vi "同步显示.vi"(8 "error in (no error)":errorcluster caption="错误输入（无错误）", 11 "程序 输入":refnum<class "程序.lvclass">) -> (0 "error out":errorcluster caption="错误输出", 3 "程序 输出":refnum<class "程序.lvclass">)   [LabVIEW 2018, in "程序.lvclass"]
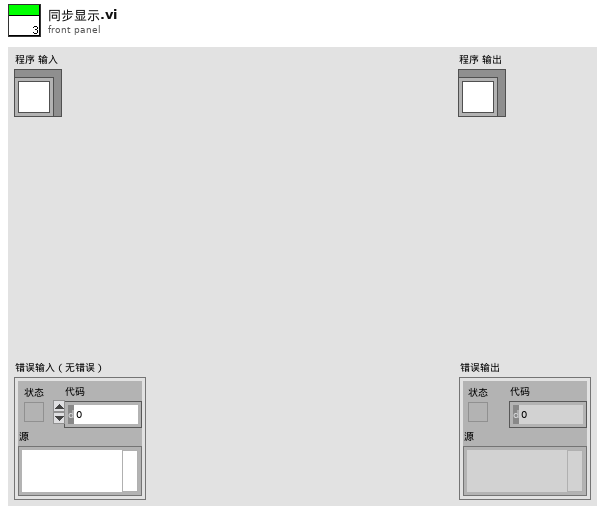
[diagram p1: front panel]
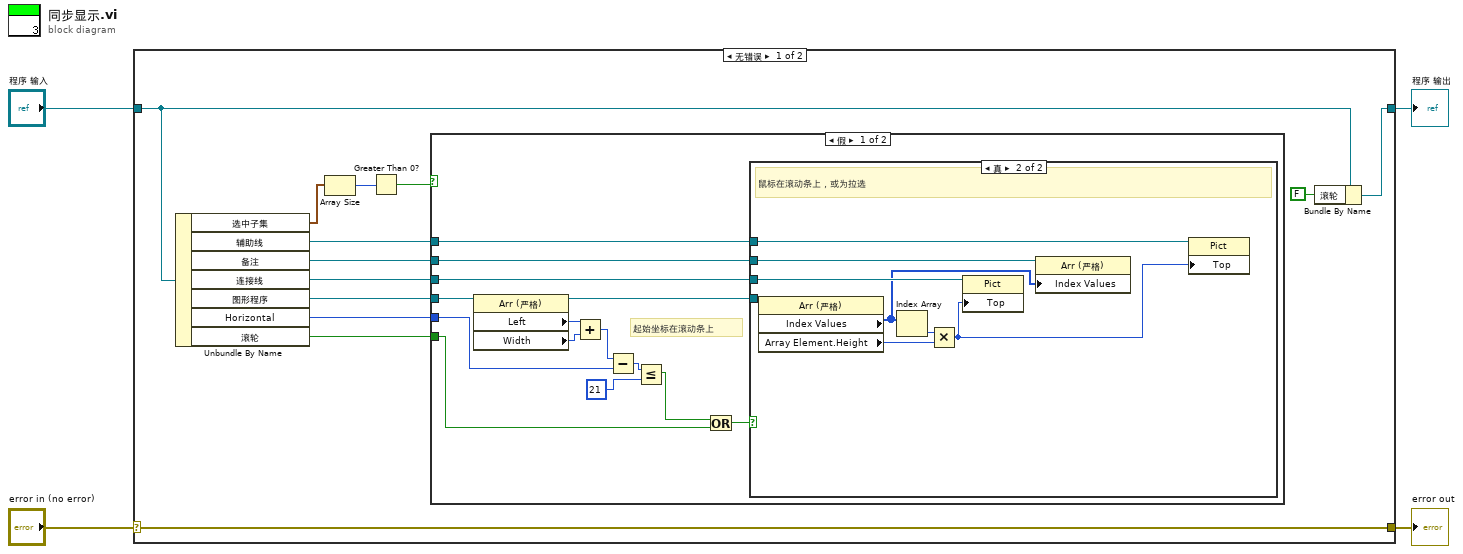
[diagram p0: block diagram]
diagram:
  n1 = case shown="无错误" "error in (no error)" {
    selector: "error in (no error)" -> [w17 w41]
    tunnel: [w17 w41] -> w3
    tunnel: [w9 w40] -> w1
    tunnel: "程序 输入" -> [w11 w40]
    frame No Error {
      n2 = Unbundle By Name(w11) -> ("选中子集"=w7:cluster{"行":i32, "列":i32}[], "辅助线"=w12:refnum<vi>, "备注"=w13:refnum<vi>, "连接线"=w16:refnum<vi>, "图形程序"=w15:refnum<vi>, "Horizontal"=w14:i32, "滚轮"=w8:bool)
      n3 = Array Size(array=w7) -> (size(s)=w6:i32)
      n4 = Greater Than 0?(x=w6) -> (x > 0?=w5:bool)
      n5 = case shown="假" w5 {
        tunnel: w16 -> [w31 _]
        tunnel: w15 -> [w28 _]
        tunnel: w14 -> [w25 _]
        tunnel: w13 -> [w22 _]
        tunnel: w12 -> [w21 _]
        tunnel: w8 -> [w20 _]
        frame False {
          # "起始坐标在滚动条上"
          n6 = property class="Arr (严格)"(reference=w28) -> (reference out=w27:refnum<vi>, "Left"=w30:i32, "Width"=w29:u32)  [unwired: 1 in, 1 out]
          n7 = Add(x=w30, y=w29) -> (x+y=w26:u32)
          n8 = Subtract(x=w26, y=w25) -> (x-y=w24:u32)
          n9 = Less Or Equal?(x=w24, y=u32 21) -> (x <= y?=w19:bool)
          n10 = Or(x=w19, y=w20) -> (x .or. y?=w23:bool)
          n11 = case shown="真" w23 {
            tunnel: w27 -> [_ w39]
            tunnel: w31 -> [_ w36]
            tunnel: w22 -> [_ w35]
            tunnel: w21 -> [_ w33]
            frame False {
            }
            frame True {
              # "鼠标在滚动条上，或为拉选"
              n12 = property class="Arr (严格)"(reference=w39) -> ("Index Values"=w34:u32[], "Array Element.Height"=w37:u32)  [unwired: 1 in, 2 out]
              n13 = Index Array(array=w34) -> (element=w38:u32)  [unwired: 1 in]
              n14 = Multiply(x=w38, y=w37) -> (x*y=w32:u32)
              n15 = property class="Pict"(reference=w36, "Top"=w32) -> ()  [unwired: 1 in, 2 out]
              n16 = property class="Arr (严格)"(reference=w35, "Index Values"=w34) -> ()  [unwired: 1 in, 2 out]
              n17 = property class="Pict"(reference=w33, "Top"=w32) -> ()  [unwired: 1 in, 2 out]
            }
          }
        }
        frame True {
        }
      }
      n18 = Bundle By Name(cluster=w11, "滚轮"=FALSE) -> (w9:refnum<class "程序.lvclass">)
    }
    frame Error {
    }
  }
  "error out" <- w3
  "程序 输出" <- w1
